vi "gu_strlen.vi"(8 "error in":errorcluster, 11 "Encoded String":T1) -> (0 "error out":errorcluster, 3 "Length":i32)   [LabVIEW 2020, in "G-Unicode.lvlib"]
uses:
  G-Unicode.lvlib
  Types/Encoded UTF-8 String.ctl
  lib/g_unicode_32.dll
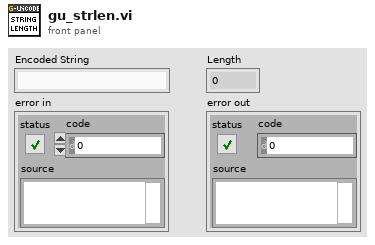
[diagram p1: front panel]
types:
  T1 = typedef "G-Unicode.lvlib/Encoded UTF-8 String.ctl" = string
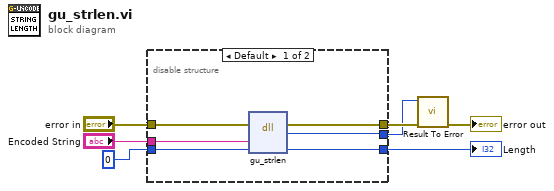
[diagram p0: block diagram]
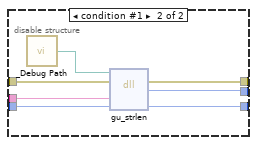
[diagram p2: hidden frame]
diagram:
  n1 = disable-structure shown="Default" {
    disable-tunnel: "Encoded String" -> [w11 w18]
    disable-tunnel: [w9 w16] -> w6
    disable-tunnel: "error in" -> [w13 w20]
    disable-tunnel: [w12 w19] -> w3
    disable-tunnel: 0 ("length") -> [w10 w15]
    disable-tunnel: [w8 w14] -> w1
    frame condition #0 (active) {
      n2 = dll-call lib="C:/github/dataflowg/g-unicode/src/LabVIEW/G-Unicode/lib/g_unicode_*.*" fn="gu_strlen"(error in=w13, "str"=w11, "length"=w10) -> (error out=w12:errorcluster, "result"=w8:i32, "length"=w9:i32)  [unwired: 3 in, 1 out]
    }
    frame condition #1 {
      n3 = call "_Debug Path.vi"() -> ("Debug Path"=w17:path)
      n4 = dll-call lib="?" fn="gu_strlen"(path in=w17, error in=w20, "str"=w18, "length"=w15) -> (error out=w19:errorcluster, "result"=w14:i32, "length"=w16:i32)  [unwired: 2 in, 1 out]
    }
  }
  "Length" <- w6
  n5 = call "Result To Error.vi"("error in (no error)"=w3, "Result Code"=w1) -> ("error out"=→"error out":errorcluster)  [unwired: 9 in]
